vi "WPI_SimpleGyro_Close.vi"(11 "SimpleGyroDevRef":T1) -> (0 "error out":errorcluster)   [LabVIEW 2014, in "SimpleGyro.lvlib"]
doc: "Closes the SimpleGyroDevRef and properly shuts down SPI communication between the RoboRIO and the SimpleGyro."
uses:
  SimpleGyro.lvlib
  WPI_SimpleGyroDevRef.ctl
  <vilib>/Rock Robotics/SystemInterfaces/Typedef/FPGA_TypedefDigitalModule.ctl
  <vilib>/Rock Robotics/SystemInterfaces/spilib/spi_bus.ctl
  <vilib>/Rock Robotics/WPI/SPI/WPI_SPIDevRef.ctl
panel:
  in  "error in":errorcluster
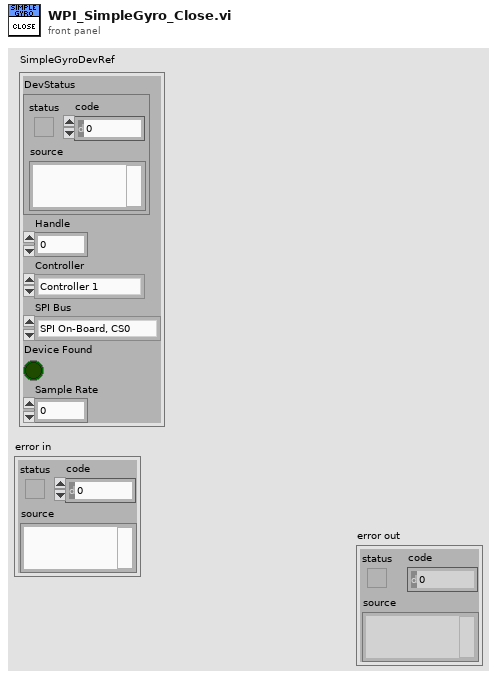
[diagram p1: front panel]
types:
  T1 = typedef "SimpleGyro.lvlib/WPI_SimpleGyroDevRef.ctl" = cluster{"DevStatus":errorcluster, "Handle":i32, "Controller":T2, "SPI Bus":T3, "Device Found":bool, "Sample Rate":dbl}
  T2 = typedef "FPGA_TypedefDigitalModule.ctl" = enum16{"Controller 1"}
  T3 = typedef "spi_bus.ctl" = enum16{"SPI On-Board, CS0", "SPI On-Board, CS1", "SPI On-Board, CS2", "SPI On-Board, CS3", "SPI MXP", "Invalid"}
  T4 = typedef "WPI_SPIDevRef.ctl" = cluster{"DevStatus":errorcluster, "Handle":i32, "Controller":T2, "SPI Bus":T3}
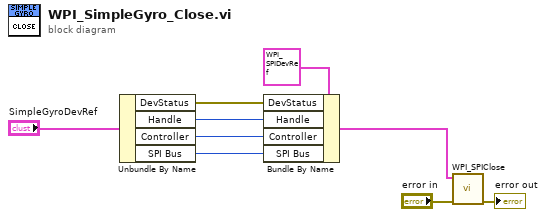
[diagram p0: block diagram]
diagram:
  n1 = Unbundle By Name("SimpleGyroDevRef") -> ("DevStatus"=w5:errorcluster, "Handle"=w4:i32, "Controller"=w3:T2, "SPI Bus"=w2:T3)
  n2 = Bundle By Name(cluster=T4 {"DevStatus"={"status"=FALSE, "code"=0, "source"=""}, "Handle"=0, "Controller"=enum."Controller 1", "SPI Bus"=enum."SPI On-Board, CS0"} ("SPIDevRef"), "DevStatus"=w5, "Handle"=w4, "Controller"=w3, "SPI Bus"=w2) -> (w1:T4)
  n3 = call <vilib>:"WPI_SPIClose.vi"("error in (no error)"="error in", "SPIDevRef"=w1) -> ("error out"=→"error out":errorcluster)  [unwired: 9 in]
